vi "CU_calcCorrelationCoeffs.vi"(8 "error in (no error)":errorcluster, 10 "Percent in":dbl, 11 "ClassifierClass in":refnum<class "ClassifierClass.lvclass">) -> (0 "error out":errorcluster, 1 "Indicies":i16[](array[numeric]), 2 "R^2 out":dbl[](array[numeric]), 3 "ClassifierClass out":refnum<class "ClassifierClass.lvclass">)   [LabVIEW 2016, in "Classifier.lvlib" / "ClassifierClass.lvclass"]
uses:
  ClassifierClass.lvclass
  ClassifierClass.lvclass/ClassifierClass.ctl
  <vilib>/gmath/statdist.llb/st_Percentiles (scalar).vi
  <vilib>/gmath/NI_Gmath.lvlib
panel:
  # "This VI is a part of BCI Design library, http://www.ru-bci.org \nCopyright © 2020, Sotnikov Peter, All rights reserved. License: CC BY-NC 4.0"
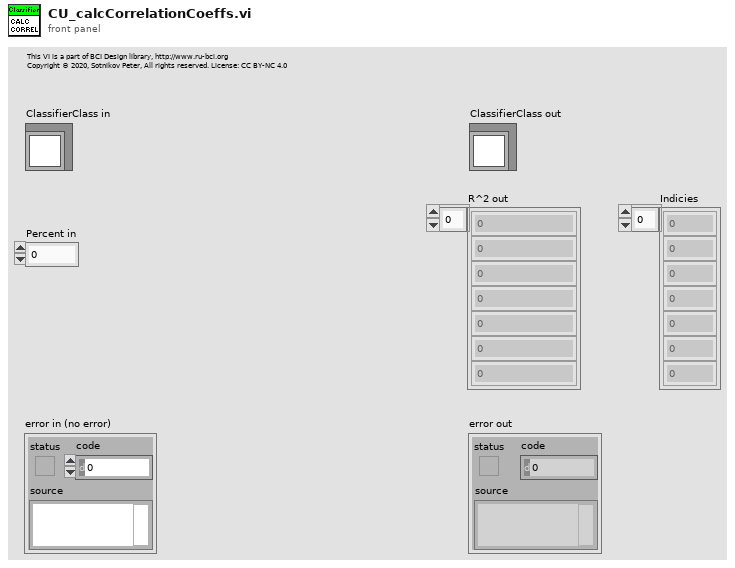
[diagram p1: front panel]
types:
  T1 = typedef "XML_EEG_Features.lvlib/XML_FF_Trial.ctl" = cluster{"ClassLabel":string, "FeatureVector":dbl[]}
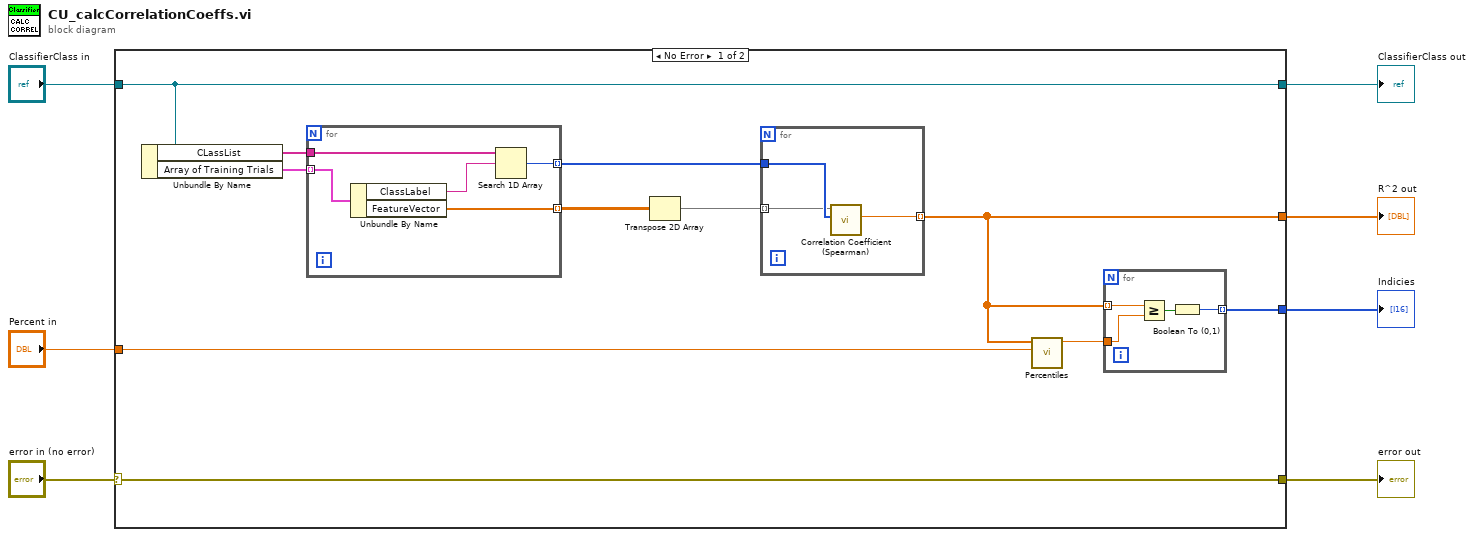
[diagram p0: block diagram]
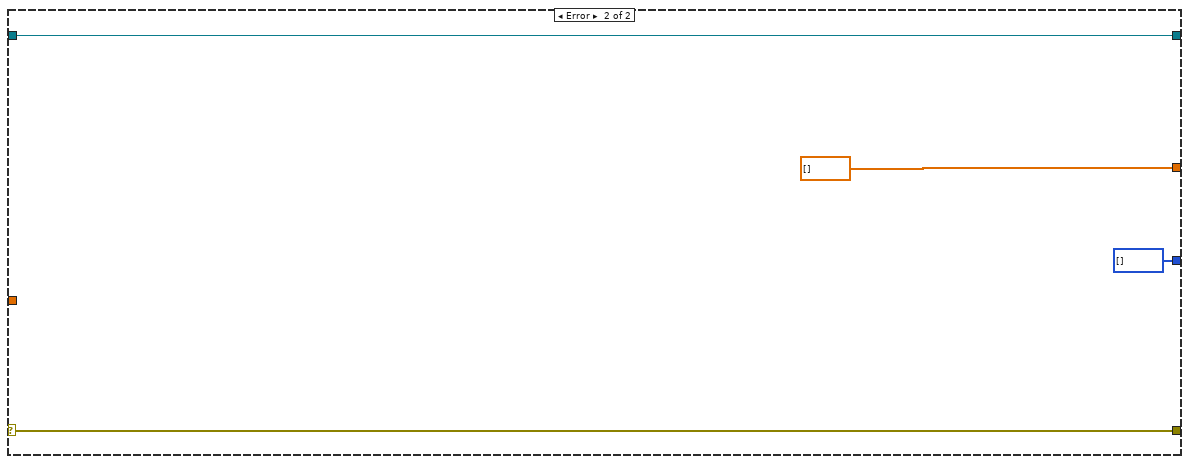
[diagram p2: hidden frame]
diagram:
  n1 = case shown="No Error" "error in (no error)" {
    selector: "error in (no error)" -> [w17 w33]
    tunnel: [w17 w33] -> w6
    tunnel: [w18 w34] -> w4
    tunnel: "ClassifierClass in" -> [w18 w34]
    tunnel: [w11 dbl[] []] -> w3
    tunnel: [w9 i16[] []] -> w2
    tunnel: "Percent in" -> [w8 _]
    frame No Error {
      n2 = Unbundle By Name(w18) -> ("CLassList"=w15:string[], "Array of Training Trials"=w16:T1[])
      n3 = for {
        tunnel: w16 -> [w30] mode=indexing
        tunnel: w15 -> [w29]
        tunnel: [w27] -> w14 mode=indexing
        tunnel: [w26] -> w13 mode=indexing
        n4 = Unbundle By Name(w30) -> ("ClassLabel"=w28:string, "FeatureVector"=w27:dbl[])
        n5 = Search 1D Array(1D array=w29, element=w28) -> (index of element=w26:i32)  [unwired: 1 in]
      }
      n6 = Transpose 2D Array(2D array=w14) -> (transposed array=w12:dbl[][])
      n7 = for {
        tunnel: w13 -> [w24]
        tunnel: w12 -> [w23] mode=indexing
        tunnel: [w25] -> w11 mode=indexing
        n8 = call <vilib>:"Correlation Coefficient (Spearman).vi"("Y"=w24, "X"=w23) -> ("r^2"=w25:dbl)  [unwired: 8 in, 1 out]
      }
      n9 = call-poly <vilib>:"Percentiles.vi"("p"=w8, "x array"=w11) -> ("percentile"=w10:dbl)  [unwired: 8 in, 1 out]
      n10 = for {
        tunnel: w11 -> [w22] mode=indexing
        tunnel: w10 -> [w21]
        tunnel: [w19] -> w9 mode=indexing
        n11 = Greater Or Equal?(x=w22, y=w21) -> (x >= y?=w20:bool)
        n12 = Boolean To (0,1)(Boolean=w20) -> (0, 1=w19:i16)
      }
    }
    frame Error {
    }
  }
  "error out" <- w6
  "ClassifierClass out" <- w4
  "R^2 out" <- w3
  "Indicies" <- w2
